vi "turn sub.vi"(7 "turn Button":bool, 8 "Stepper 1 error in":errorcluster, 9 "Stepper 1 in":T1, 10 "Pin 12 error in":errorcluster, 11 "Pin 12 in":T1) -> (0 "Stepper 1 error out":errorcluster, 1 "Stepper 1 out":T1, 2 "Pin 12 error out":errorcluster, 3 "Pin 12 out":T1)   [LabVIEW 2018]
uses:
  <vilib>/LabVIEW Interface for Arduino/Type Defs/Arduino Resource.ctl
  <vilib>/LabVIEW Interface for Arduino/Type Defs/Board Type.ctl
  <vilib>/LabVIEW Interface for Arduino/LabVIEW Interface for Arduino.lvlib
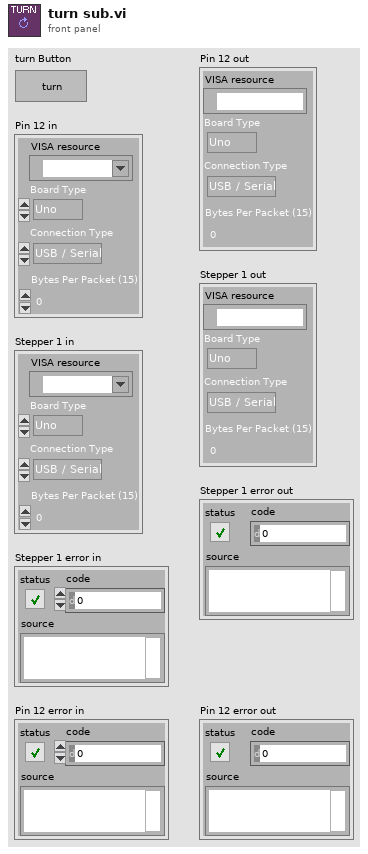
[diagram p1: front panel]
types:
  T1 = typedef "LabVIEW Interface for Arduino.lvlib/Arduino Resource.ctl" = cluster{"VISA resource":refnum<visa-resource-name>, "Board Type":T2, "Connection Type":enum8{"USB / Serial"}, "Bytes Per Packet (15)":u8}
  T2 = typedef "LabVIEW Interface for Arduino.lvlib/Board Type.ctl" = enum16{"Uno", "Dimuelanove w/Atmega 328", "Mega 2560"}
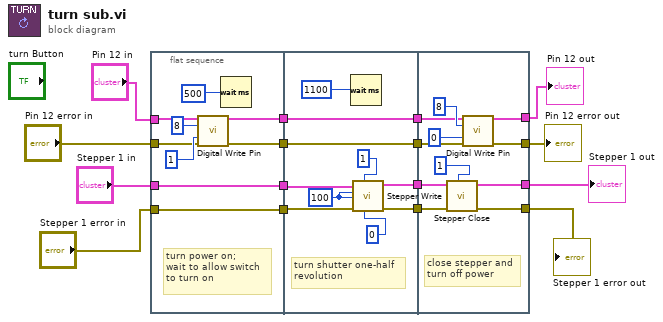
[diagram p0: block diagram]
diagram:
  n1 = flat-sequence {
    tunnel: "Stepper 1 in" -> [w19]
    tunnel: "Stepper 1 error in" -> [w18]
    tunnel: [w19] -> w16
    tunnel: [w18] -> w15
    tunnel: "Pin 12 in" -> [w23]
    tunnel: "Pin 12 error in" -> [w22]
    tunnel: [w21] -> w14
    tunnel: [w20] -> w13
    tunnel: w16 -> [w32]
    tunnel: w15 -> [w33]
    tunnel: [w31] -> w12
    tunnel: [w30] -> w11
    tunnel: [w29] -> w10
    tunnel: w14 -> [w29]
    tunnel: [w28] -> w9
    tunnel: w13 -> [w28]
    tunnel: w12 -> [w38]
    tunnel: w11 -> [w39]
    tunnel: [w36] -> w3
    tunnel: [w40] -> w4
    tunnel: w10 -> [w44]
    tunnel: w9 -> [w43]
    tunnel: [w42] -> w7
    tunnel: [w41] -> w8
    frame #0 {
      # "turn power on;\nwait to allow switch\nto turn on"
      n2 = call <vilib>:"Digital Write Pin.vi"("Arduino Resource"=w23, "Digital I/O Pin (0)"=8, "Value (0)"=1, "error in"=w22) -> ("Arduino Resource"=w21:T1, "error out"=w20:errorcluster)  [unwired: 10 in]
      n3 = Wait (ms)(milliseconds to wait=500) -> ()  [unwired: 1 out]
    }
    frame #1 {
      w26 = 100
      # "turn shutter one-half\nrevolution"
      n4 = Wait (ms)(milliseconds to wait=1100) -> ()  [unwired: 1 out]
      n5 = call <vilib>:"Stepper Write.vi"("Set Acceleration (0 to disable)"=0, "Stepper #"=1, "error in"=w33, "Set Speed (Steps per Second)"=w26, "# of Steps to Move"=w26, "Arduino Resource"=w32) -> ("error out"=w31:errorcluster, "Arduino Resource Out"=w30:T1)  [unwired: 4 in]
    }
    frame #2 {
      # "close stepper and\nturn off power"
      n6 = call <vilib>:"Stepper Close.vi"("Stepper #"=1, "error in"=w38, "Arduino Resource"=w39) -> ("error out"=w40:errorcluster, "Arduino Resource Out"=w36:T1)  [unwired: 7 in]
      n7 = call <vilib>:"Digital Write Pin.vi"("Arduino Resource"=w44, "Digital I/O Pin (0)"=8, "Value (0)"=0, "error in"=w43) -> ("Arduino Resource"=w42:T1, "error out"=w41:errorcluster)  [unwired: 10 in]
    }
  }
  "Pin 12 error out" <- w8
  "Pin 12 out" <- w7
  "Stepper 1 error out" <- w4
  "Stepper 1 out" <- w3
